vi "RFmx_Meas_Settings_Defaults.vi"(8 "error in":errorcluster, 10 "Measurements":T1(array[ring]), 11 "Instrument Handle in":refnum<k21>) -> (0 "error out":errorcluster, 1 "Selector_Strings":string[](array[string]), 3 "Instrument Handle out":refnum<k21>)   [LabVIEW 2014]
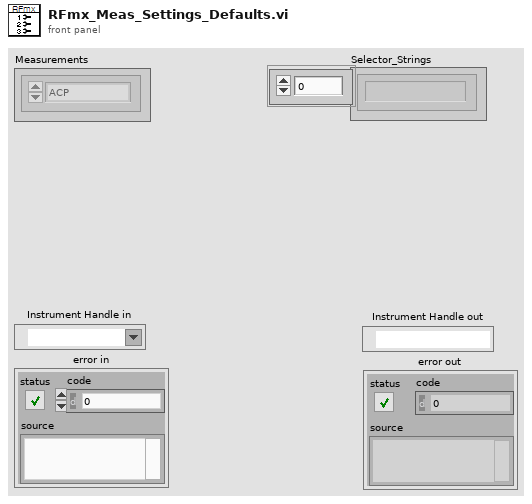
[diagram p1: front panel]
types:
  T1 = enum16{"ACP", "CCDF", "CHP", "FCnt", "Harmonics", "OBW", "SEM", "Spectrum", "Spur", "TXP", "AMPM", "DPD", "IQ"}[]
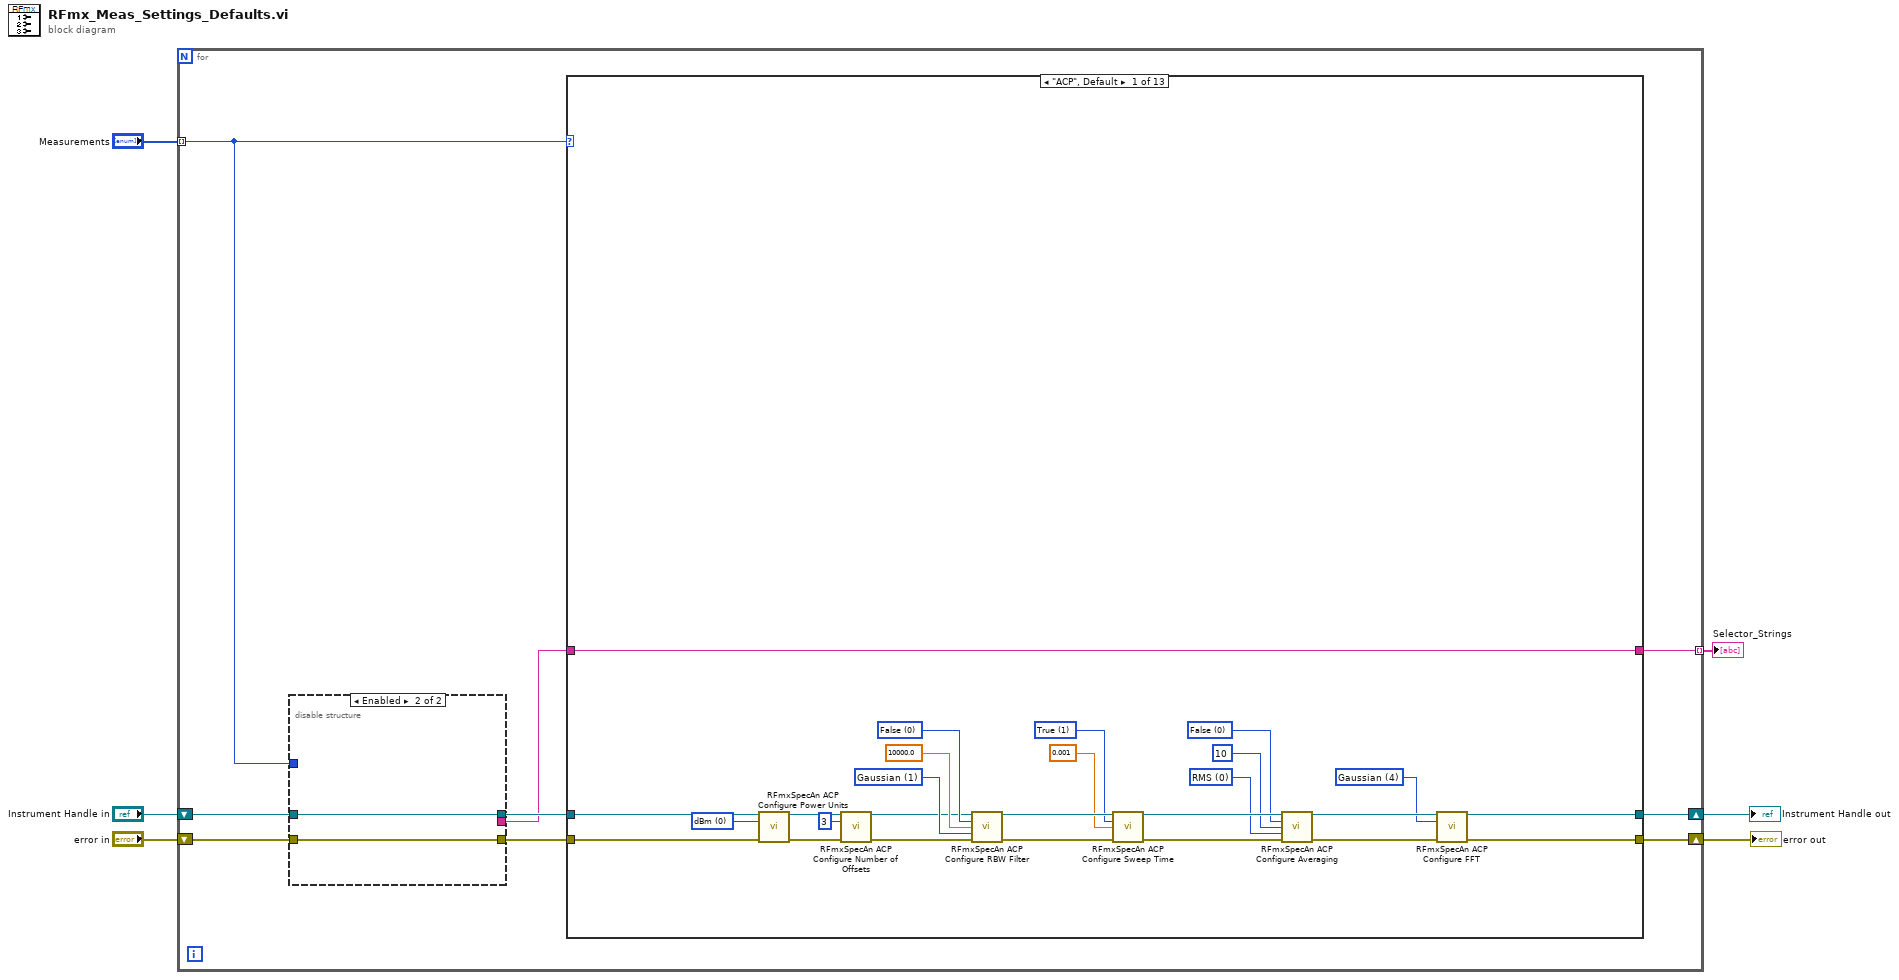
[diagram p0: block diagram]
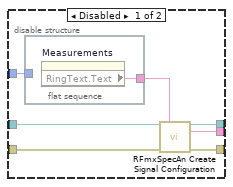
[diagram p2: hidden frame]
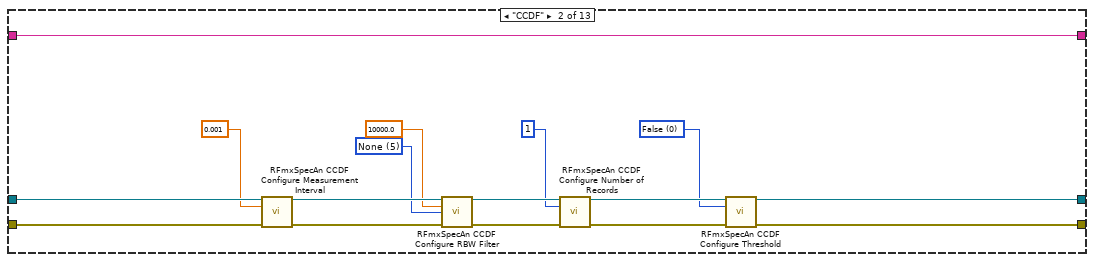
[diagram p3: hidden frame]
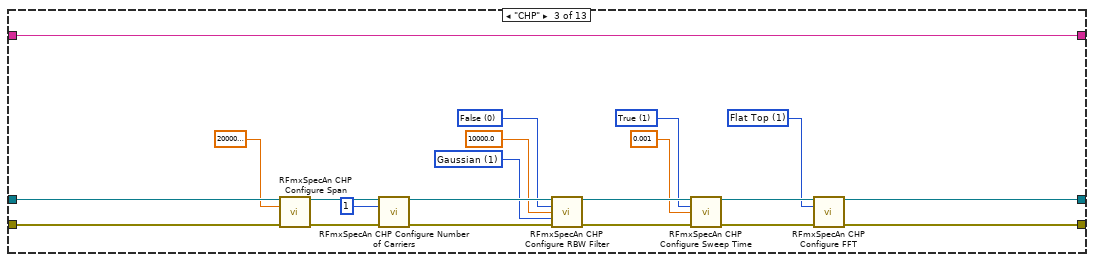
[diagram p4: hidden frame]
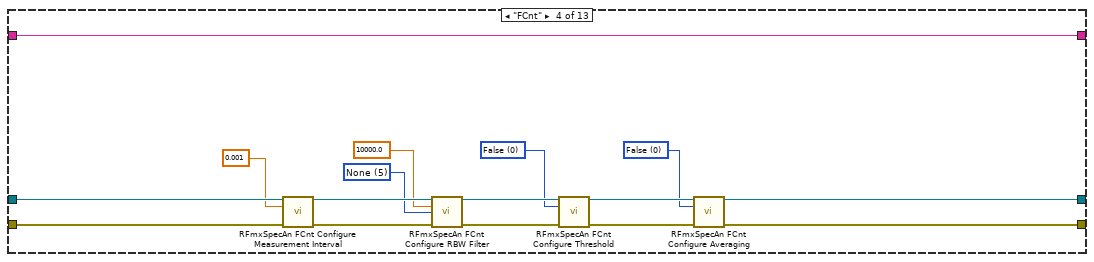
[diagram p5: hidden frame]
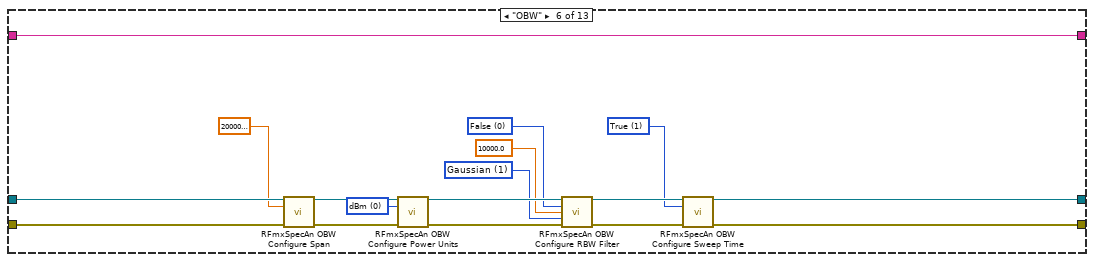
[diagram p7: hidden frame]
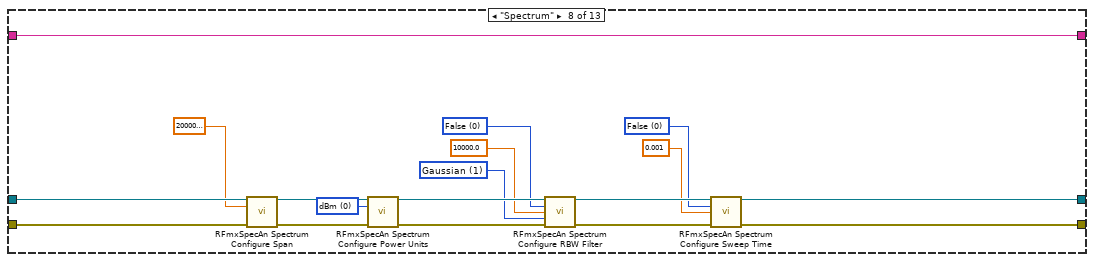
[diagram p9: hidden frame]
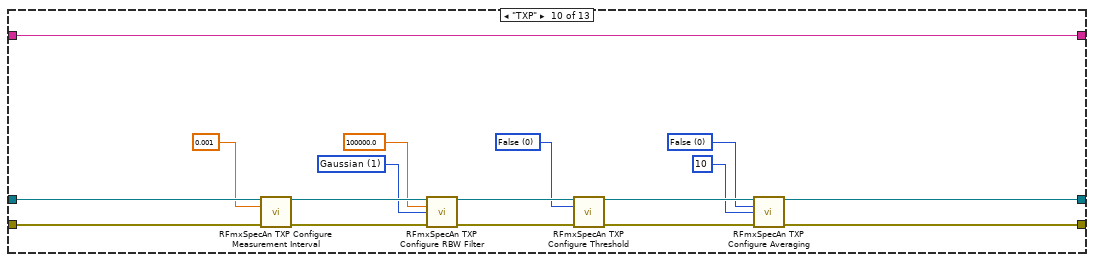
[diagram p11: hidden frame]
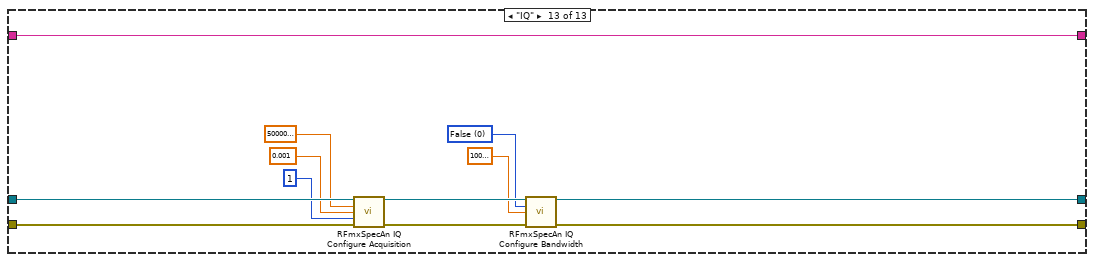
[diagram p14: hidden frame]
diagram:
  n1 = for {
    shift-right: [w15] -> w6
    shift-left: "Instrument Handle in" -> [w13]
    shift-right: [w14] -> w5
    shift-left: "error in" -> [w12]
    tunnel: "Measurements" -> [w8] mode=indexing
    tunnel: [w7] -> w1 mode=indexing
    n2 = disable-structure shown="Enabled" {
      disable-tunnel: w13 -> [w21 w25]
      disable-tunnel: w12 -> [w20 w24]
      disable-tunnel: [w19 w24] -> w11
      disable-tunnel: [w18 w25] -> w10
      disable-tunnel: [w17 _] -> w9
      disable-tunnel: w8 -> [w16 _]
      frame Disabled {
        n3 = flat-sequence {
          tunnel: w16 -> [_]
          tunnel: [w23] -> w22
          frame #0 {
            n4 = property on="Measurements" class="Enum (strict)"() -> ("RingText.Text"=w23:string)  [unwired: 2 in, 2 out]
          }
        }
        n5 = call <vilib>:"RFmxSpecAn Create Signal Configuration.vi"("Instrument Handle In"=w21, "Signal Name"=w22, "error in (no error)"=w20) -> ("Instrument Handle Out"=w18:refnum<k21>, "Selector String Out"=w17:string, "error out"=w19:errorcluster)  [unwired: 10 in]
      }
      frame Enabled {
      }
    }
    n6 = case shown="\"ACP\", Default" w8 {
      tunnel: w10 -> [w51 w67 w88 w104 w106 w124 w127 w145 w148 w165 w168 w171 w183]
      tunnel: w11 -> [w50 w66 w87 w103 w107 w123 w126 w144 w147 w164 w167 w170 w182]
      tunnel: [w32 w55 w70 w91 w106 w110 w127 w130 w148 w154 w168 w171 w176] -> w15
      tunnel: [w31 w54 w69 w90 w107 w109 w126 w129 w147 w153 w167 w170 w175] -> w14
      tunnel: w9 -> [w33 w52 w68 w89 w105 w108 w125 w128 w146 w149 w166 w169 w172]
      tunnel: [w33 w52 w68 w89 w105 w108 w125 w128 w146 w149 w166 w169 w172] -> w7
      frame "ACP", Default {
        w35 = 1 items=["False", "True"] ("Sweep Time Auto")
        w36 = 0 items=["RMS", "Log", "Scalar", "Max", "Min", "Vector"] ("Averaging Type")
        w38 = 0 items=["False", "True"] ("Averaging Enabled")
        w39 = 4 items=["None", "Flat Top", "Hanning", "Hamming", "Gaussian", "Blackman", "Blackman-Harris", "Kaiser-Bessel"] ("FFT Window")
        w46 = 1 items=["FFT Based", "Gaussian", "Flat", "Synch Tuned - 4", "Synch Tuned - 5"] ("RBW Filter Type")
        w48 = 0 items=["False", "True"] ("RBW Auto")
        w49 = 0 items=["dBm", "dBm/Hz"] ("Power Units")
        n7 = call <vilib>:"RFmxSpecAn ACP Configure Power Units.vi"("Instrument Handle In"=w51, "Power Units"=w49, "error in (no error)"=w50) -> ("Instrument Handle Out"=w30:refnum<k21>, "error out"=w29:errorcluster)  [unwired: 11 in]
        n8 = call <vilib>:"RFmxSpecAn ACP Configure Number of Offsets.vi"("Instrument Handle In"=w30, "Number of Offsets"=3, "error in (no error)"=w29) -> ("Instrument Handle Out"=w28:refnum<k21>, "error out"=w27:errorcluster)  [unwired: 11 in]
        n9 = call <vilib>:"RFmxSpecAn ACP Configure RBW Filter.vi"("Instrument Handle In"=w28, "RBW Auto"=w48, "RBW (Hz)"=10000.0, "RBW Filter Type"=w46, "error in (no error)"=w27) -> ("Instrument Handle Out"=w45:refnum<k21>, "error out"=w44:errorcluster)  [unwired: 9 in]
        n10 = call <vilib>:"RFmxSpecAn ACP Configure Sweep Time.vi"("Instrument Handle In"=w45, "Sweep Time Auto"=w35, "Sweep Time Interval (s)"=0.001, "error in (no error)"=w44) -> ("Instrument Handle Out"=w43:refnum<k21>, "error out"=w42:errorcluster)  [unwired: 10 in]
        n11 = call <vilib>:"RFmxSpecAn ACP Configure Averaging.vi"("Instrument Handle In"=w43, "Averaging Enabled"=w38, "Averaging Count"=10, "Averaging Type"=w36, "error in (no error)"=w42) -> ("Instrument Handle Out"=w41:refnum<k21>, "error out"=w40:errorcluster)  [unwired: 9 in]
        n12 = call <vilib>:"RFmxSpecAn ACP Configure FFT.vi"("Instrument Handle In"=w41, "FFT Window"=w39, "error in (no error)"=w40) -> ("Instrument Handle Out"=w32:refnum<k21>, "error out"=w31:errorcluster)  [unwired: 11 in]
      }
      frame "CCDF" {
        w56 = 0 items=["False", "True"] ("Threshold Enabled")
        w62 = 5 items=["None"=5, "Gaussian"=1, "Flat"=2, "Synch Tuned - 4"=3, "Synch Tuned - 5"=4, "RRC"=6] ("RBW Filter Type")
        n13 = call <vilib>:"RFmxSpecAn CCDF Configure Measurement Interval.vi"("Instrument Handle In"=w67, "Measurement Interval (s)"=0.001, "error in (no error)"=w66) -> ("Instrument Handle Out"=w65:refnum<k21>, "error out"=w64:errorcluster)  [unwired: 11 in]
        n14 = call <vilib>:"RFmxSpecAn CCDF Configure RBW Filter.vi"("Instrument Handle In"=w65, "RBW (Hz)"=10000.0, "RBW Filter Type"=w62, "error in (no error)"=w64) -> ("Instrument Handle Out"=w61:refnum<k21>, "error out"=w60:errorcluster)  [unwired: 10 in]
        n15 = call <vilib>:"RFmxSpecAn CCDF Configure Number of Records.vi"("Instrument Handle In"=w61, "Number of Records"=1, "error in (no error)"=w60) -> ("Instrument Handle Out"=w58:refnum<k21>, "error out"=w57:errorcluster)  [unwired: 11 in]
        n16 = call <vilib>:"RFmxSpecAn CCDF Configure Threshold.vi"("Instrument Handle In"=w58, "Threshold Enabled"=w56, "error in (no error)"=w57) -> ("Instrument Handle Out"=w55:refnum<k21>, "error out"=w54:errorcluster)  [unwired: 11 in]
      }
      frame "CHP" {
        w71 = 1 items=["None", "Flat Top", "Hanning", "Hamming", "Gaussian", "Blackman", "Blackman-Harris", "Kaiser-Bessel"] ("FFT Window")
        w75 = 1 items=["False", "True"] ("Sweep Time Auto")
        w78 = 1 items=["FFT Based", "Gaussian", "Flat", "Synch Tuned - 4", "Synch Tuned - 5"] ("RBW Filter Type")
        w80 = 0 items=["False", "True"] ("RBW Auto")
        n17 = call <vilib>:"RFmxSpecAn CHP Configure Span.vi"("Instrument Handle In"=w88, "Span (Hz)"=20000000.0, "error in (no error)"=w87) -> ("Instrument Handle Out"=w84:refnum<k21>, "error out"=w83:errorcluster)  [unwired: 11 in]
        n18 = call <vilib>:"RFmxSpecAn CHP Configure Number of Carriers.vi"("Instrument Handle In"=w84, "Number of Carriers"=1, "error in (no error)"=w83) -> ("Instrument Handle Out"=w82:refnum<k21>, "error out"=w81:errorcluster)  [unwired: 11 in]
        n19 = call <vilib>:"RFmxSpecAn CHP Configure RBW Filter.vi"("Instrument Handle In"=w82, "RBW Auto"=w80, "RBW (Hz)"=10000.0 ("Span (Hz)"), "RBW Filter Type"=w78, "error in (no error)"=w81) -> ("Instrument Handle Out"=w77:refnum<k21>, "error out"=w76:errorcluster)  [unwired: 9 in]
        n20 = call <vilib>:"RFmxSpecAn CHP Configure Sweep Time.vi"("Instrument Handle In"=w77, "Sweep Time Auto"=w75, "Sweep Time Interval (s)"=0.001, "error in (no error)"=w76) -> ("Instrument Handle Out"=w73:refnum<k21>, "error out"=w72:errorcluster)  [unwired: 10 in]
        n21 = call <vilib>:"RFmxSpecAn CHP Configure FFT.vi"("Instrument Handle In"=w73, "FFT Window"=w71, "error in (no error)"=w72) -> ("Instrument Handle Out"=w70:refnum<k21>, "error out"=w69:errorcluster)  [unwired: 11 in]
      }
      frame "FCnt" {
        w93 = 0 items=["False", "True"] ("Averaging Enabled")
        w95 = 0 items=["False", "True"] ("Threshold Enabled")
        w98 = 5 items=["None"=5, "Gaussian"=1, "Flat"=2, "Synch Tuned - 4"=3, "Synch Tuned - 5"=4, "RRC"=6] ("RBW Filter Type")
        n22 = call <vilib>:"RFmxSpecAn FCnt Configure Measurement Interval.vi"("Instrument Handle In"=w104, "Measurement Interval (s)"=0.001, "error in (no error)"=w103) -> ("Instrument Handle Out"=w101:refnum<k21>, "error out"=w100:errorcluster)  [unwired: 11 in]
        n23 = call <vilib>:"RFmxSpecAn FCnt Configure RBW Filter.vi"("Instrument Handle In"=w101, "RBW (Hz)"=10000.0, "RBW Filter Type"=w98, "error in (no error)"=w100) -> ("Instrument Handle Out"=w97:refnum<k21>, "error out"=w96:errorcluster)  [unwired: 10 in]
        n24 = call <vilib>:"RFmxSpecAn FCnt Configure Threshold.vi"("Instrument Handle In"=w97, "Threshold Enabled"=w95, "error in (no error)"=w96) -> ("Instrument Handle Out"=w94:refnum<k21>, "error out"=w92:errorcluster)  [unwired: 11 in]
        n25 = call <vilib>:"RFmxSpecAn FCnt Configure Averaging.vi"("Instrument Handle In"=w94, "Averaging Enabled"=w93, "error in (no error)"=w92) -> ("Instrument Handle Out"=w91:refnum<k21>, "error out"=w90:errorcluster)  [unwired: 11 in]
      }
      frame "Harmonics" {
        # "Harmonics는 5665, 5668R에만 적용 가능함"
      }
      frame "OBW" {
        w111 = 1 items=["False", "True"] ("Sweep Time Auto")
        w114 = 1 items=["FFT Based", "Gaussian", "Flat", "Synch Tuned - 4", "Synch Tuned - 5"] ("RBW Filter Type")
        w116 = 0 items=["False", "True"] ("RBW Auto")
        w119 = 0 items=["dBm", "dBm/Hz"] ("Power Units")
        n26 = call <vilib>:"RFmxSpecAn OBW Configure Span.vi"("Instrument Handle In"=w124, "Span (Hz)"=20000000.0, "error in (no error)"=w123) -> ("Instrument Handle Out"=w121:refnum<k21>, "error out"=w120:errorcluster)  [unwired: 11 in]
        n27 = call <vilib>:"RFmxSpecAn OBW Configure Power Units.vi"("Instrument Handle In"=w121, "Power Units"=w119, "error in (no error)"=w120) -> ("Instrument Handle Out"=w118:refnum<k21>, "error out"=w117:errorcluster)  [unwired: 11 in]
        n28 = call <vilib>:"RFmxSpecAn OBW Configure RBW Filter.vi"("Instrument Handle In"=w118, "RBW Auto"=w116, "RBW (Hz)"=10000.0, "RBW Filter Type"=w114, "error in (no error)"=w117) -> ("Instrument Handle Out"=w113:refnum<k21>, "error out"=w112:errorcluster)  [unwired: 9 in]
        n29 = call <vilib>:"RFmxSpecAn OBW Configure Sweep Time.vi"("Instrument Handle In"=w113, "Sweep Time Auto"=w111, "error in (no error)"=w112) -> ("Instrument Handle Out"=w110:refnum<k21>, "error out"=w109:errorcluster)  [unwired: 11 in]
      }
      frame "SEM" {
        # "적용해야할 부분이 많으므로 다음에 추가할 예정"
      }
      frame "Spectrum" {
        w132 = 0 items=["False", "True"] ("Sweep Time Auto")
        w135 = 1 items=["FFT Based", "Gaussian", "Flat", "Synch Tuned - 4", "Synch Tuned - 5"] ("RBW Filter Type")
        w137 = 0 items=["False", "True"] ("RBW Auto")
        w141 = 0 items=["dBm", "dBm/Hz", "dBW", "dBV", "dBmV", "dBuV", "W", "Volts", "Volts Squared"] ("Power Units")
        n30 = call <vilib>:"RFmxSpecAn Spectrum Configure Span.vi"("Instrument Handle In"=w145, "Span (Hz)"=20000000.0, "error in (no error)"=w144) -> ("Instrument Handle Out"=w142:refnum<k21>, "error out"=w140:errorcluster)  [unwired: 11 in]
        n31 = call <vilib>:"RFmxSpecAn Spectrum Configure Power Units.vi"("Instrument Handle In"=w142, "Power Units"=w141, "error in (no error)"=w140) -> ("Instrument Handle Out"=w139:refnum<k21>, "error out"=w138:errorcluster)  [unwired: 11 in]
        n32 = call <vilib>:"RFmxSpecAn Spectrum Configure RBW Filter.vi"("Instrument Handle In"=w139, "RBW Auto"=w137, "RBW (Hz)"=10000.0, "RBW Filter Type"=w135, "error in (no error)"=w138) -> ("Instrument Handle Out"=w134:refnum<k21>, "error out"=w133:errorcluster)  [unwired: 9 in]
        n33 = call <vilib>:"RFmxSpecAn Spectrum Configure Sweep Time.vi"("Instrument Handle In"=w134, "Sweep Time Auto"=w132, "Sweep Time Interval (s)"=0.001, "error in (no error)"=w133) -> ("Instrument Handle Out"=w130:refnum<k21>, "error out"=w129:errorcluster)  [unwired: 10 in]
      }
      frame "Spur" {
        # "Spur는 5665, 5668R에만 적용 가능함"
      }
      frame "TXP" {
        w151 = 0 items=["False", "True"] ("Averaging Enabled")
        w157 = 0 items=["False", "True"] ("Threshold Enabled")
        w159 = 1 items=["None"=5, "Gaussian"=1, "Flat"=2, "Synch Tuned - 4"=3, "Synch Tuned - 5"=4, "RRC"=6] ("RBW Filter Type")
        n34 = call <vilib>:"RFmxSpecAn TXP Configure Measurement Interval.vi"("Instrument Handle In"=w165, "Measurement Interval (s)"=0.001, "error in (no error)"=w164) -> ("Instrument Handle Out"=w162:refnum<k21>, "error out"=w161:errorcluster)  [unwired: 11 in]
        n35 = call <vilib>:"RFmxSpecAn TXP Configure RBW Filter.vi"("Instrument Handle In"=w162, "RBW (Hz)"=100000.0, "RBW Filter Type"=w159, "error in (no error)"=w161) -> ("Instrument Handle Out"=w158:refnum<k21>, "error out"=w156:errorcluster)  [unwired: 10 in]
        n36 = call <vilib>:"RFmxSpecAn TXP Configure Threshold.vi"("Instrument Handle In"=w158, "Threshold Enabled"=w157, "error in (no error)"=w156) -> ("Instrument Handle Out"=w155:refnum<k21>, "error out"=w152:errorcluster)  [unwired: 11 in]
        n37 = call <vilib>:"RFmxSpecAn TXP Configure Averaging.vi"("Instrument Handle In"=w155, "Averaging Enabled"=w151, "Averaging Count"=10, "error in (no error)"=w152) -> ("Instrument Handle Out"=w154:refnum<k21>, "error out"=w153:errorcluster)  [unwired: 10 in]
      }
      frame "AMPM" {
        # "적용해야할 부분이 많으므로 다음에 추가할 예정"
      }
      frame "DPD" {
        # "적용해야할 부분이 많으므로 다음에 추가할 예정"
      }
      frame "IQ" {
        w174 = 0 items=["False", "True"] ("Bandwidth Auto")
        n38 = call <vilib>:"RFmxSpecAn IQ Configure Acquisition.vi"("Instrument Handle In"=w183, "Sample Rate (S/s)"=50000000.0, "Acquisition Time (s)"=0.001, "Number of Records"=1, "error in (no error)"=w182) -> ("Instrument Handle Out"=w178:refnum<k21>, "error out"=w177:errorcluster)  [unwired: 9 in]
        n39 = call <vilib>:"RFmxSpecAn IQ Configure Bandwidth.vi"("Instrument Handle In"=w178, "Bandwidth Auto"=w174, "Bandwidth (Hz)"=1000000.0, "error in (no error)"=w177) -> ("Instrument Handle Out"=w176:refnum<k21>, "error out"=w175:errorcluster)  [unwired: 10 in]
      }
    }
  }
  "Instrument Handle out" <- w6
  "error out" <- w5
  "Selector_Strings" <- w1
